vi "wr_rd_ser.vi"(3 "error in":errorcluster, 4 "string to write":string, 5 "VISA resource name in":refnum<visa-resource-name>) -> (0 "error out":errorcluster, 1 "read buffer":string, 2 "VISA resource name out":refnum<visa-resource-name>)   [LabVIEW 2009]
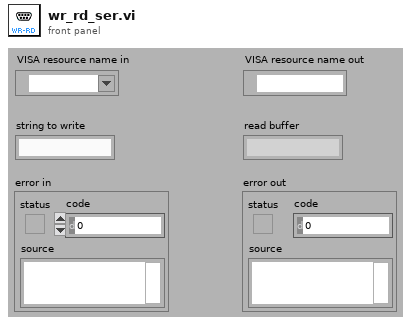
[diagram p1: front panel]
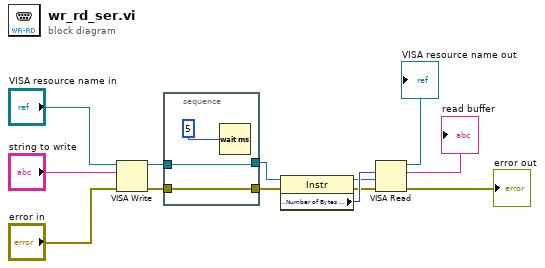
[diagram p0: block diagram]
diagram:
  n1 = VISA Write(VISA resource name="VISA resource name in", write buffer="string to write", error in (no error)="error in") -> (VISA resource name out=w4:refnum<visa-resource-name>, error out=w5:errorcluster)  [unwired: 1 out]
  n2 = stacked-sequence {
    tunnel: w4 -> [w15]
    tunnel: w5 -> [w14]
    tunnel: [w15] -> w12
    tunnel: [w14] -> w13
    frame #0 {
      n3 = Wait (ms)(milliseconds to wait=u32 5 ("delay before read (ms)")) -> ()  [unwired: 1 out]
    }
  }
  n4 = property class="Instr"(reference=w12, error in=w13) -> (reference out=w6:refnum<visa-resource-name>, error out=w7:errorcluster, "Serial Settings:Number of Bytes at Serial Port"=w8:u32)
  n5 = VISA Read(VISA resource name=w6, byte count=w8, error in (no error)=w7) -> (VISA resource name out=→"VISA resource name out":refnum<visa-resource-name>, read buffer=→"read buffer":string, error out=→"error out":errorcluster)  [unwired: 1 out]
